vi "Measurement Logic.vi"(8 "error in":errorcluster, 9 "measurement configuration":T2={"Automation Test"=FALSE, "Power sequencing file path"="", "RFmx name"="5842_0", "RFmx port"="", "DUT Max Gain (dB)"=2.0, "DUT Max Noise Figure (dB)"=2.0, "Reference Level Mode"=enum."Manual", "Reference Level (dBm)"=2.0, "Preamp Enabled"=1, "RFmx attenuation mode"=enum."Constant Attenuation", "RFmx external attenuation (dB)"=1.2, "RFmx s-parameters orientation"=enum."Port2 Towards DUT", "RFmx s2p file path"="", "Switch Name"="", "Switch Connection"="", "ENS SMU Name"="", "ENS SMU Channel"="", "Action"=0, "Measurement Bandwidth (Hz)"=4000000.0, "Measurement Interval (s)"=0.1, "NF Cal Setup ID"="SNS_PS_6dB_ENR15_26.5GHz_VI", "DUT Type"=0, "Frequency List Mode"=enum."Step", "Step - Start Frequency "=1000000000.0, "Step - Stop Frequency"=2000000000.0, "Step - Step Size"=100000000.0, "Points - Start Frequency"=1000000000.0, "Points - Stop Frequency"=2000000000.0, "Points - Number of Points"=11, "FreqList - Frequency List"=[4000000000.0, 5000000000.0, 6000000000.0, 7000000000.0, 8000000000.0, 9000000000.0, 10000000000.0, 11000000000.0, 12000000000.0, 13000000000.0, 14000000000.0, 15000000000.0, 16000000000.0, 17000000000.0, 18000000000.0, 19000000000.0, 20000000000.0], "Averaging Enabled"=FALSE, "Averaging Count"=10, "Noise Source Type"=1, "Noise Source RFSG Port"="port1", "Noise Source Cold Temperature (K)"=302.8, "Noise Source Off Temperature (K)"=297.0, "ENR Freq (Hz)"=[6500000000.0], "ENR (dB)"=[15.0], "DUT Input_Compensation Enabled"=FALSE, "DUT Input_Temperation (K)"=297.0, "DUT Input_Loss Freq (Hz)"=array[589 elements], "DUT Input_Loss (dB)"=array[589 elements], "DUT Output_Compensation Enabled"=FALSE, "DUT Output_Temperation (K)"=297.0, "DUT Output_Loss Freq (Hz)"=array[589 elements], "DUT Output_Loss (dB)"=array[589 elements], "Calibration_Compensation Enabled"=FALSE, "Calibration_Temperation (K)"=297.0, "Calibration_Loss Freq (Hz)"=array[589 elements], "Calibration_Loss (dB)"=array[589 elements], "Noise Source_Compensation Enabled"=FALSE, "Noise Source_Temperation (K)"=297.0, "Noise Source_Loss Freq (Hz)"=[], "Noise Source_Loss (dB)"=[], "DUT Input Loss S2P File Path"="", "DUT Input Loss S-Parameter Orientation"=0, "DUT Output Loss S2P File Path"="", "DUT Output Loss S-Parameter Orientation"=0, "Calibration Loss S2P File Path"="", "Calibration Loss S-Parameter Orientation"=0, "Noise Source Loss S2P File Path"="", "Noise Source Loss S-Parameter Orientation"=0} {"Noise Source Loss S-Parameter Orientation" items=["Port1 Towards DUT", "Port2 Towards DUT"]; "Calibration Loss S-Parameter Orientation" items=["Port1 Towards DUT", "Port2 Towards DUT"]; "DUT Output Loss S-Parameter Orientation" items=["Port1 Towards DUT", "Port2 Towards DUT"]; "DUT Input Loss S-Parameter Orientation" items=["Port1 Towards DUT", "Port2 Towards DUT"]; "FreqList - Frequency List" format="%.3p Hz"; "Points - Stop Frequency" format="%.3p Hz"; "Points - Start Frequency" format="%.3p Hz"; "Step - Step Size" format="%.3p Hz"; "Step - Stop Frequency" format="%.3p Hz"; "Step - Start Frequency" format="%.3p Hz"; "Noise Source_Loss (dB)" format="%.2g"; "Noise Source_Loss Freq (Hz)" format="%.3p"; "Noise Source_Temperation (K)" format="%.2g"; "Calibration_Loss (dB)" format="%.2g"; "Calibration_Loss Freq (Hz)" format="%.3p"; "Calibration_Temperation (K)" format="%.2g"; "DUT Output_Loss (dB)" format="%.2g"; "DUT Output_Loss Freq (Hz)" format="%.3p"; "DUT Output_Temperation (K)" format="%.2g"; "DUT Input_Loss (dB)" format="%.2g"; "DUT Input_Loss Freq (Hz)" format="%.3p"; "DUT Input_Temperation (K)" format="%.2g"; "ENR (dB)" format="%.2g"; "ENR Freq (Hz)" format="%.3p"; "Noise Source Off Temperature (K)" format="%.2f"; "Noise Source Cold Temperature (K)" format="%.2f"; "Noise Source Type" items=["External Noise Source", "RF Signal Generator"]; "DUT Type" items=["Amplifier", "Downconverter", "Upconverter"]; "Measurement Interval (s)" format="%.2p"; "Measurement Bandwidth (Hz)" format="%.3p"; "Action" items=["Measure", "Calibrate"]; "RFmx external attenuation (dB)" format="%.2f"; "Preamp Enabled" items=["Disabled"=0, "Enabled"=1, "Automatic"=3]}, 10 "measure call context in":refnum<class "Measure Call Context.lvclass">) -> (0 "error out":errorcluster, 1 "measurement results":T1 {"Analyzer NF (mean)" format="%.2g"; "DUT NF (mean)" format="%.2g"; "Analyzer NF vs Freq" format="%.2g"; "DUT NF vs Freq" format="%.2g"}, 2 "measure call context out":refnum<class "Measure Call Context.lvclass">)   [LabVIEW 2023, in "FPT NoiseFigure.lvclass"]
doc: "Contains the core logic for executing the measurement."
uses:
  FPT NoiseFigure.lvclass
  <vilib>/Plug-In SDKs/Measurements/Measure Call Context/Measure Call Context.lvclass
  Measurement Configuration.ctl
  Measurement Results.ctl
  <vilib>/Analysis/baseanly.llb/Mean (DBL).vi
  <extravilib>/ChannelInstances/Event Messenger-bool/Instantiate.vi
  <vilib>/Analysis/NI_AALBase.lvlib
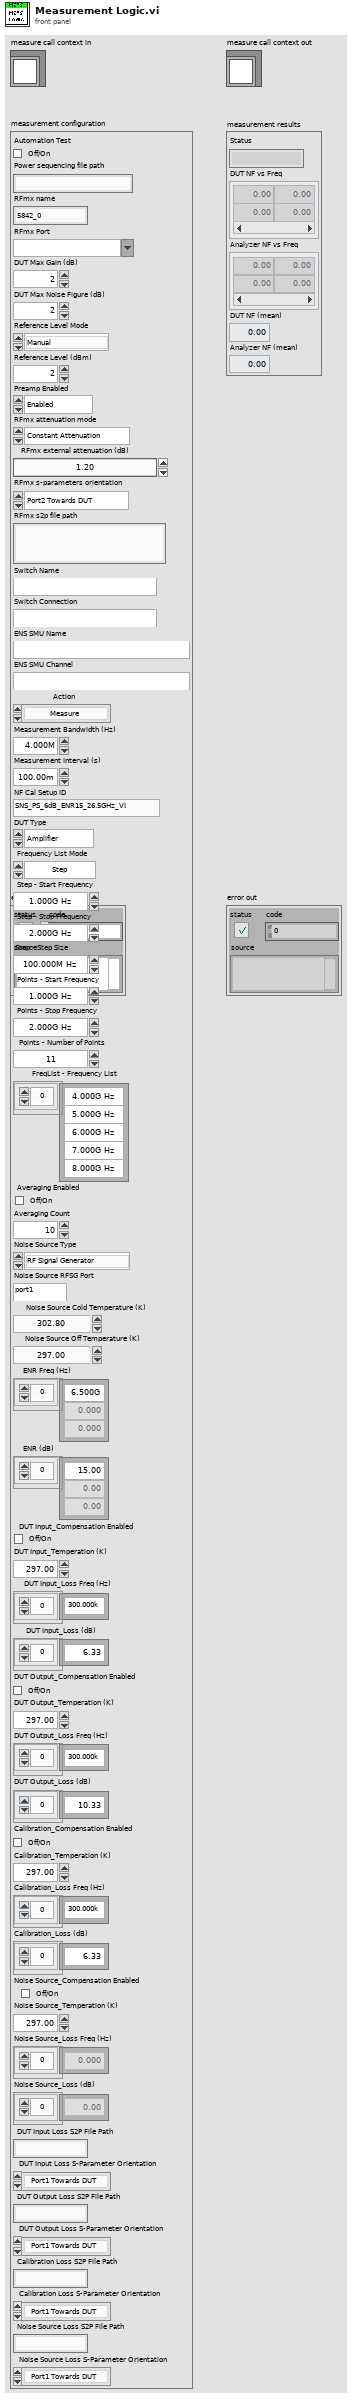
[diagram p1: front panel]
types:
  T1 = typedef "FPT NoiseFigure.lvclass/Measurement Results.ctl" = cluster{"Status":string, "DUT NF vs Freq":dbl[][], "Analyzer NF vs Freq":dbl[][], "DUT NF (mean)":dbl, "Analyzer NF (mean)":dbl}
  T2 = typedef "FPT NoiseFigure.lvclass/Measurement Configuration.ctl" = cluster{"Automation Test":bool, "Power sequencing file path":string, "RFmx name":string, "RFmx port":string, "DUT Max Gain (dB)":dbl, "DUT Max Noise Figure (dB)":dbl, "Reference Level Mode":enum32{"Manual", "Recommend"}, "Reference Level (dBm)":dbl, "Preamp Enabled":i32, "RFmx attenuation mode":enum32{"<None>", "Constant Attenuation", "s2p File"}, "RFmx external attenuation (dB)":dbl, "RFmx s-parameters orientation":enum32{"Port1 Towards DUT", "Port2 Towards DUT"}, "RFmx s2p file path":string, "Switch Name":string, "Switch Connection":string, "ENS SMU Name":string, "ENS SMU Channel":string, "Action":u32, "Measurement Bandwidth (Hz)":dbl, "Measurement Interval (s)":dbl, "NF Cal Setup ID":string, "DUT Type":i32, "Frequency List Mode":enum32{"Step", "Points", "Frequency List"}, "Step - Start Frequency ":dbl, "Step - Stop Frequency":dbl, "Step - Step Size":dbl, "Points - Start Frequency":dbl, "Points - Stop Frequency":dbl, "Points - Number of Points":i32, "FreqList - Frequency List":dbl[], "Averaging Enabled":bool, "Averaging Count":i32, "Noise Source Type":i32, "Noise Source RFSG Port":string, "Noise Source Cold Temperature (K)":dbl, "Noise Source Off Temperature (K)":dbl, "ENR Freq (Hz)":dbl[], "ENR (dB)":dbl[], "DUT Input_Compensation Enabled":bool, "DUT Input_Temperation (K)":dbl, "DUT Input_Loss Freq (Hz)":dbl[], "DUT Input_Loss (dB)":dbl[], "DUT Output_Compensation Enabled":bool, "DUT Output_Temperation (K)":dbl, "DUT Output_Loss Freq (Hz)":dbl[], "DUT Output_Loss (dB)":dbl[], "Calibration_Compensation Enabled":bool, "Calibration_Temperation (K)":dbl, "Calibration_Loss Freq (Hz)":dbl[], "Calibration_Loss (dB)":dbl[], "Noise Source_Compensation Enabled":bool, "Noise Source_Temperation (K)":dbl, "Noise Source_Loss Freq (Hz)":dbl[], "Noise Source_Loss (dB)":dbl[], "DUT Input Loss S2P File Path":string, "DUT Input Loss S-Parameter Orientation":i32, "DUT Output Loss S2P File Path":string, "DUT Output Loss S-Parameter Orientation":i32, "Calibration Loss S2P File Path":string, "Calibration Loss S-Parameter Orientation":i32, "Noise Source Loss S2P File Path":string, "Noise Source Loss S-Parameter Orientation":i32}
  T3 = enum32{"Power On Dut", "De-embedding + Measurement", "Power Off Dut"}[]
  T4 = cluster{"measurement configuration":T2, "measurement results":T1}
  T5 = typedef "RFmx Config - NF.ctl" = cluster{"RFmx Name":refnum<k15>, "RFmx Port":string, "Reference Level":cluster{"DUT Max Gain (dB)":dbl, "DUT Max Noise Figure (dB)":dbl, "Mode":enum32{"Manual", "Recommend"}, "Reference Level (dBm)":dbl}, "Preamp Enabled":i32, "Attenuation":cluster{"Mode":enum32{"<None>", "Constant Attenuation", "s2p File"}, "Constant Attenuation":cluster{"RFmx External Attenuation (dB)":dbl}, "s2p File":cluster{"RFmx S-Parameters Orientation":i32, "RFmx Attenuation s2p File":path}}, "ENS Source":cluster{"SMU Name":refnum<k15>, "SMU Channel":string}}
  T6 = typedef "Test Config - NF.ctl" = cluster{"Y-Factor Mode":i32, "Measurement Bandwidth (Hz)":dbl, "Measurement Interval (s)":dbl, "NF Cal Setup ID":string, "NF DUT Type":i32, "Frequency List (Hz)":dbl[], "Averaging":cluster{"Enabled":i32, "Count":i32}, "Noise Source":cluster{"Noise Source Type":i32, "Noise Source RFSG Port":string, "Cold Temperature (K)":dbl, "Off Temperature (K)":dbl, "ENR Freq (Hz)":dbl[], "ENR (dB)":dbl[]}}
  T7 = typedef "Switches - NF.ctl" = cluster{"Switch Name":refnum<k15>, "Connection":string}
  T8 = typedef "Path Loss Settings Cluster.ctl" = cluster{"DUT Input Loss":T9, "DUT Output Loss":T9, "Calibration Loss":T9, "Noise Source Loss":T9}
  T9 = typedef "Path Loss Settings.ctl" = cluster{"Compensation Enabled":i32, "Temperation (K)":dbl, "S2P Path":path, "Orientation":enum32{"Port1 Towards DUT", "Port2 Towards DUT"}}
  T10 = typedef "Event Messenger-bool.lvlib/))Channel.ctl" = refnum<queue>
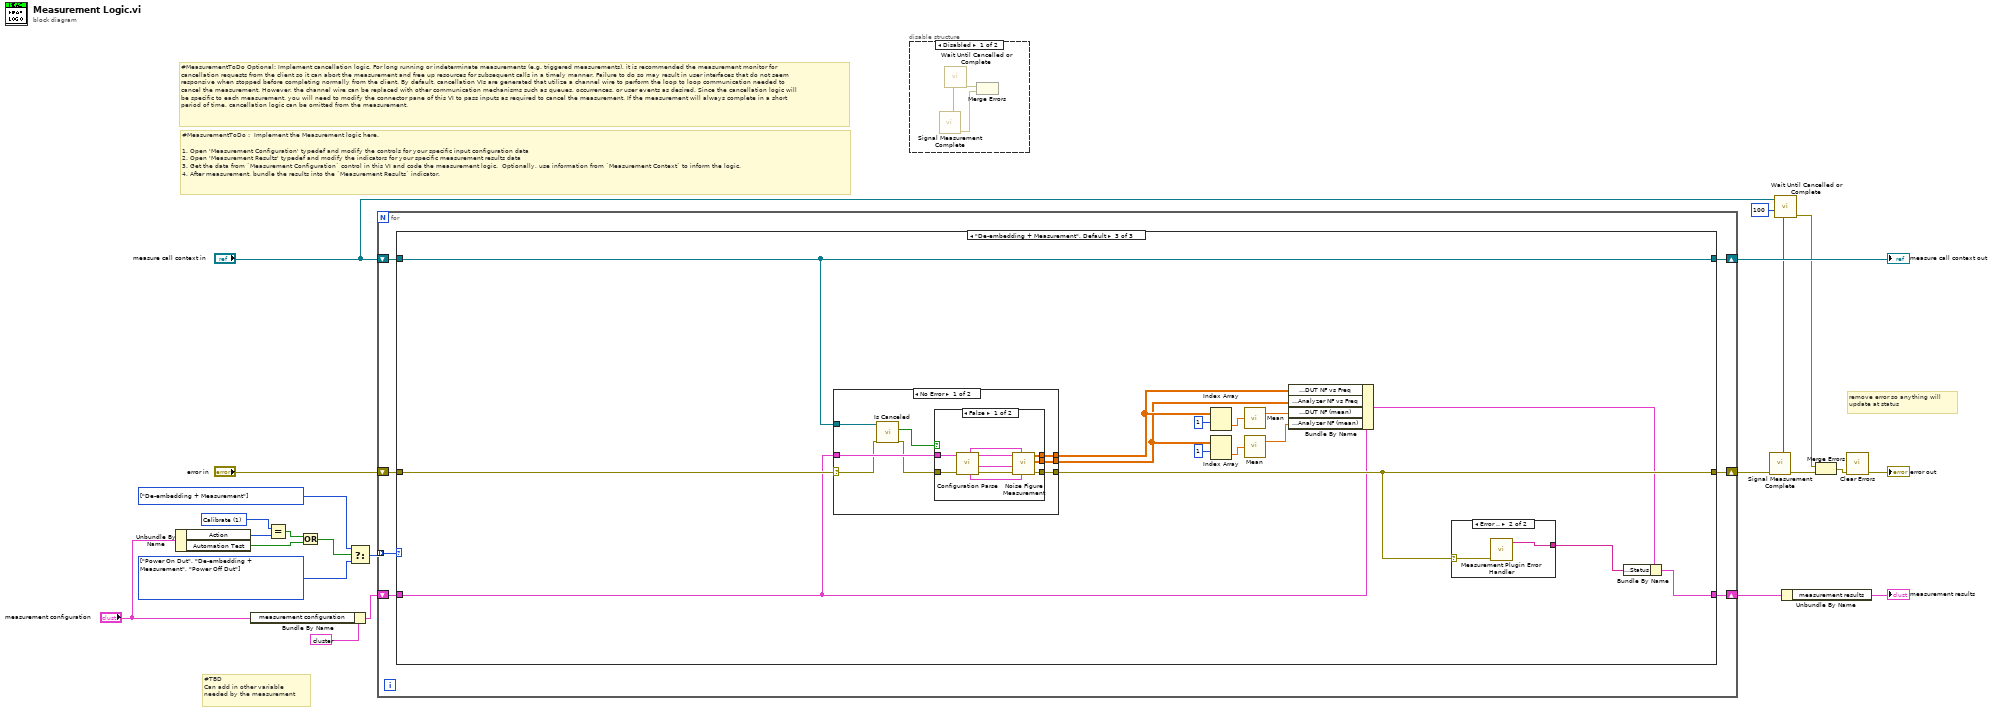
[diagram p0: block diagram]
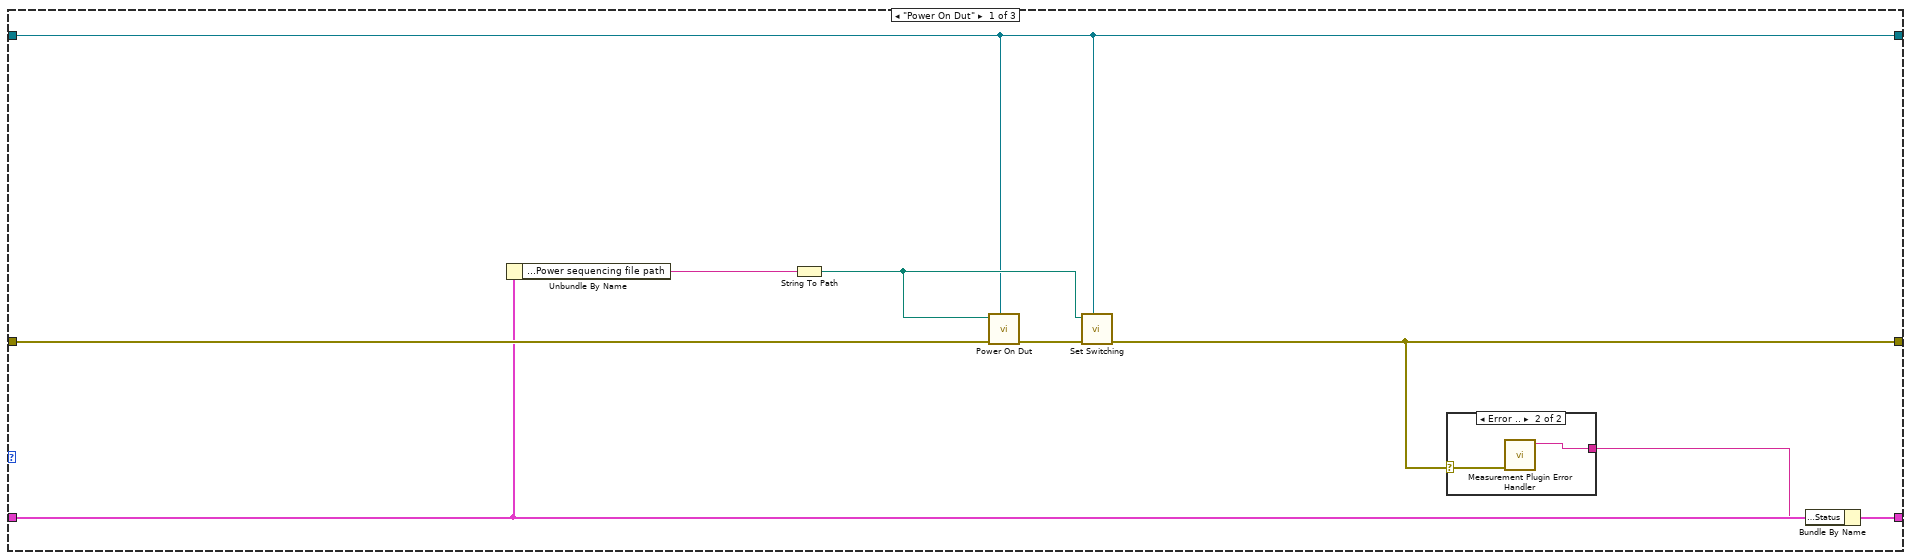
[diagram p2: hidden frame]
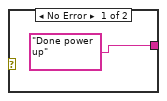
[diagram p3: hidden frame]
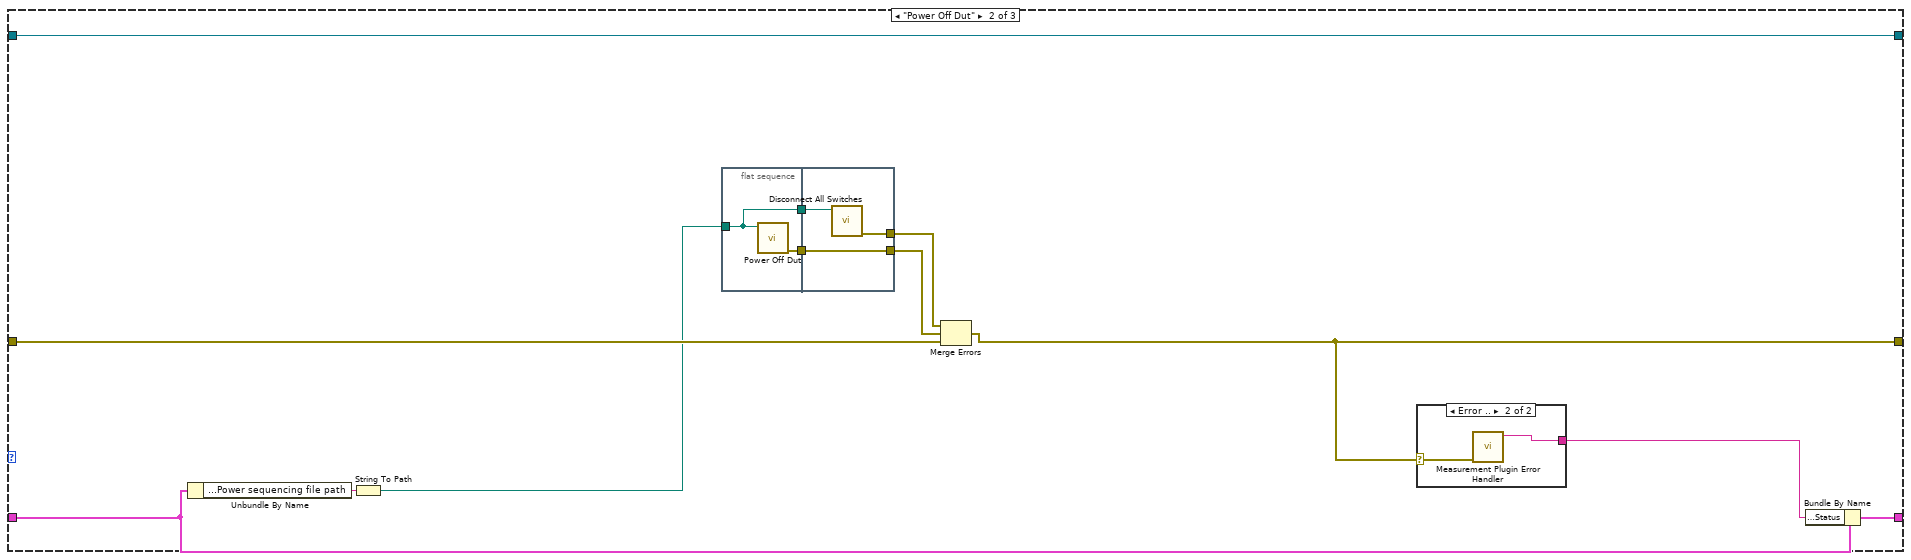
[diagram p4: hidden frame]
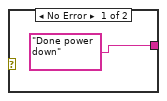
[diagram p5: hidden frame]
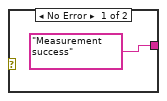
[diagram p6: hidden frame]
diagram:
  w8 = u32 1 items=["Measure", "Calibrate"] ("Y-Factor Mode")
  w15 = T3 [enum."De-embedding + Measurement"] items=["Power On Dut", "De-embedding + Measurement", "Power Off Dut"]
  w16 = T3 [enum."Power On Dut", enum."De-embedding + Measurement", enum."Power Off Dut"] items=["Power On Dut", "De-embedding + Measurement", "Power Off Dut"]
  # "remove error so anything will\nupdate at status"
  # "#TBD\nCan add in other variable\nneeded by the measurement"
  # "#MeasurementToDo Optional: Implement cancellation logic. For long running or indeterminate measurements (e.g. triggered measurements), it is recommended the measurement monitor for cancellation requests from the client so it can abort the measurement and free up resources for subsequent calls in a timely manner. Failure to do so may result in user interfaces that do not seem responsive when stopped before completing normally from the client. By default, cancellation VIs are generated that utilize a channel wire to perform the loop to loop communication needed to cancel the measurement. However, the channel wire can be replaced with other communication mechanisms such as queues, occurrences, or user events as desired. Since the cancellation logic will be specific to each measurement, you will need to modify the connector pane of this VI to pass inputs as required to cancel the measurement. If the measurement will always complete in a short period of time, cancellation logic can be omitted from the measurement."
  # "#MeasurementToDo :  Implement the Measurement logic here.\n\n1. Open 'Measurement Configuration' typedef and modify the controls for your specific input configuration data\n2. Open 'Measurement Results' typedef and modify the indicators for your specific measurement results data\n3. Get the data from `Measurement Configuration` control in this VI and code the measurement logic.  Optionally, use information from `Measurement Context` to inform the logic.\n4. After measurement, bundle the results into the `Measurement Results` indicator."
  n1 = Unbundle By Name("measurement configuration") -> ("Action"=w13:u32, "Automation Test"=w11:bool)
  n2 = Bundle By Name(cluster=T4 {"measurement configuration"={"Automation Test"=FALSE, "Power sequencing file path"="", "RFmx name"="5842_0", "RFmx port"="", "DUT Max Gain (dB)"=2.0, "DUT Max Noise Figure (dB)"=2.0, "Reference Level Mode"=enum."Manual", "Reference Level (dBm)"=2.0, "Preamp Enabled"=1, "RFmx attenuation mode"=enum."Constant Attenuation", "RFmx external attenuation (dB)"=1.2, "RFmx s-parameters orientation"=enum."Port2 Towards DUT", "RFmx s2p file path"="", "Switch Name"="", "Switch Connection"="", "ENS SMU Name"="", "ENS SMU Channel"="", "Action"=0, "Measurement Bandwidth (Hz)"=4000000.0, "Measurement Interval (s)"=0.1, "NF Cal Setup ID"="SNS_PS_6dB_ENR15_26.5GHz_VI", "DUT Type"=0, "Frequency List Mode"=enum."Step", "Step - Start Frequency "=1000000000.0, "Step - Stop Frequency"=2000000000.0, "Step - Step Size"=100000000.0, "Points - Start Frequency"=1000000000.0, "Points - Stop Frequency"=2000000000.0, "Points - Number of Points"=11, "FreqList - Frequency List"=[4000000000.0, 5000000000.0, 6000000000.0, 7000000000.0, 8000000000.0, 9000000000.0, 10000000000.0, 11000000000.0, 12000000000.0, 13000000000.0, 14000000000.0, 15000000000.0, 16000000000.0, 17000000000.0, 18000000000.0, 19000000000.0, 20000000000.0], "Averaging Enabled"=FALSE, "Averaging Count"=10, "Noise Source Type"=1, "Noise Source RFSG Port"="port1", "Noise Source Cold Temperature (K)"=302.8, "Noise Source Off Temperature (K)"=297.0, "ENR Freq (Hz)"=[6500000000.0], "ENR (dB)"=[15.0], "DUT Input_Compensation Enabled"=FALSE, "DUT Input_Temperation (K)"=297.0, "DUT Input_Loss Freq (Hz)"=array[589 elements], "DUT Input_Loss (dB)"=array[589 elements], "DUT Output_Compensation Enabled"=FALSE, "DUT Output_Temperation (K)"=297.0, "DUT Output_Loss Freq (Hz)"=array[589 elements], "DUT Output_Loss (dB)"=array[589 elements], "Calibration_Compensation Enabled"=FALSE, "Calibration_Temperation (K)"=297.0, "Calibration_Loss Freq (Hz)"=array[589 elements], "Calibration_Loss (dB)"=array[589 elements], "Noise Source_Compensation Enabled"=FALSE, "Noise Source_Temperation (K)"=297.0, "Noise Source_Loss Freq (Hz)"=[], "Noise Source_Loss (dB)"=[], "DUT Input Loss S2P File Path"="", "DUT Input Loss S-Parameter Orientation"=0, "DUT Output Loss S2P File Path"="", "DUT Output Loss S-Parameter Orientation"=0, "Calibration Loss S2P File Path"="", "Calibration Loss S-Parameter Orientation"=0, "Noise Source Loss S2P File Path"="", "Noise Source Loss S-Parameter Orientation"=0}, "measurement results"={"Status"="", "DUT NF vs Freq"=[], "Analyzer NF vs Freq"=[], "DUT NF (mean)"=0.0, "Analyzer NF (mean)"=0.0}}, "measurement configuration"="measurement configuration") -> (w21:T4)
  n3 = Equal?(x=w8, y=w13) -> (x = y?=w14:bool)
  n4 = Or(x=w14, y=w11) -> (x .or. y?=w12:bool)
  n5 = Select(t=w15, s=w12, f=w16) -> (s? t:f=w10:T3)
  n6 = for {
    tunnel: w10 -> [w29] mode=indexing
    shift-right: [w24] -> w5
    shift-left: "error in" -> [w30]
    shift-right: [w25] -> w19
    shift-left: w21 -> [w28]
    shift-right: [w26] -> w20
    shift-left: "measure call context in" -> [w27]
    n7 = case shown="\"De-embedding + Measurement\", Default" w29 {
      tunnel: w30 -> [w39 w49 w65]
      tunnel: w28 -> [w38 w50 w64]
      tunnel: w27 -> [w31 w53 w63]
      tunnel: [w33 w48 w75] -> w24
      tunnel: [w31 w53 w63] -> w26
      tunnel: [w36 w51 w76] -> w25
      frame "Power On Dut" {
        n8 = Unbundle By Name(w38) -> ("measurement configuration.Power sequencing file path"=w35:string)
        n9 = String To Path(string=w35) -> (path=w32:path)
        n10 = call "Power On Dut.vi"("measure call context in"=w31, "error in"=w39, "Power sequencing file path"=w32) -> ("error out"=w34:errorcluster)  [unwired: 7 in, 1 out]
        n11 = call "Set Switching.vi"("measure call context in"=w31, "error in"=w34, "File Path"=w32) -> ("error out"=w33:errorcluster)  [unwired: 7 in, 1 out]
        n12 = case shown="Error .." w33 {
          selector: w33 -> [_ w42]
          tunnel: ["Done power up" w41] -> w37
          frame No Error {
          }
          frame Error {
            n13 = call "Measurement Plugin Error Handler.vi"("error in"=w42) -> ("Status Message (Error)"=w41:string)  [unwired: 9 in, 1 out]
          }
        }
        n14 = Bundle By Name(cluster=w38, "measurement results.Status"=w37) -> (w36:T4)
      }
      frame "Power Off Dut" {
        n15 = Unbundle By Name(w50) -> ("measurement configuration.Power sequencing file path"=w54:string)
        n16 = String To Path(string=w54) -> (path=w45:path)
        n17 = flat-sequence {
          tunnel: w45 -> [w58]
          tunnel: [w59] -> w47
          tunnel: [w58] -> w46
          tunnel: [w62] -> w44
          tunnel: w47 -> [w62]
          tunnel: [w61] -> w43
          tunnel: w46 -> [w60]
          frame #0 {
            n18 = call "Power Off Dut.vi"("Power Sequencing File Path"=w58) -> ("error out"=w59:errorcluster)  [unwired: 10 in]
          }
          frame #1 {
            n19 = call "Disconnect All Switches.vi"("File Path"=w60) -> ("error out"=w61:errorcluster)  [unwired: 10 in]
          }
        }
        n20 = Merge Errors(w43, w44, w49) -> (w48:errorcluster)
        n21 = case shown="Error .." w48 {
          selector: w48 -> [_ w57]
          tunnel: ["Done power down" w56] -> w52
          frame No Error {
          }
          frame Error {
            n22 = call "Measurement Plugin Error Handler.vi"("error in"=w57) -> ("Status Message (Error)"=w56:string)  [unwired: 9 in, 1 out]
          }
        }
        n23 = Bundle By Name(cluster=w50, "measurement results.Status"=w52) -> (w51:T4)
      }
      frame "De-embedding + Measurement", Default {
        n24 = case shown="No Error" w65 {
          selector: w65 -> [w83 w100]
          tunnel: [w88 w100] -> w75
          tunnel: [w87 _] -> w67
          tunnel: [w86 _] -> w66
          tunnel: w64 -> [w85 _]
          tunnel: w63 -> [w82 _]
          frame No Error {
            n25 = call <vilib>:"Is Canceled.vi"("error in"=w83, "measure call context in"=w82) -> ("error out"=w84:errorcluster, "is canceled?"=w81:bool)  [unwired: 7 in, 1 out]
            n26 = case shown="False" w81 {
              tunnel: [w98 w99] -> w88
              tunnel: [w93 _] -> w87
              tunnel: [w92 _] -> w86
              tunnel: w85 -> [w90 _]
              tunnel: w84 -> [w89 w99]
              frame False {
                n27 = call "Configuration Parse.vi"("error in"=w89, "UI Controls"=w90) -> ("error out"=w94:errorcluster, "RFmx Settings"=w96:T5, "Test Configuration"=w97:T6, "Switch"=w91:T7, "Path Losses"=w95:T8)  [unwired: 5 in]
                n28 = call "Noise Figure Measurement.vi"("Switch"=w91, "Path Losses"=w95, "error in"=w94, "RFmx Settings"=w96, "Test Configuration"=w97) -> ("error out"=w98:errorcluster, "Analyzer Noise Figure (dB)"=w92:dbl[][], "DUT Noise Figure (dB)"=w93:dbl[][])  [unwired: 3 in, 1 out]
              }
              frame True {
              }
            }
          }
          frame Error {
          }
        }
        n29 = Index Array(array=w67, index (row)=1) -> (element=w72:dbl[])  [unwired: 1 in]
        n30 = Index Array(array=w66, index (row)=1) -> (element=w71:dbl[])  [unwired: 1 in]
        n31 = call-poly <vilib>:"Mean.vi"("X"=w72) -> ("mean"=w69:dbl)  [unwired: 1 out]
        n32 = call-poly <vilib>:"Mean.vi"("X"=w71) -> ("mean"=w68:dbl)  [unwired: 1 out]
        n33 = Bundle By Name(cluster=w64, "measurement results.DUT NF vs Freq"=w67, "measurement results.Analyzer NF vs Freq"=w66, "measurement results.DUT NF (mean)"=w69, "measurement results.Analyzer NF (mean)"=w68) -> (w74:T4)
        n34 = case shown="Error .." w75 {
          selector: w75 -> [_ w80]
          tunnel: ["Measurement success" w79] -> w77
          frame No Error {
          }
          frame Error {
            n35 = call "Measurement Plugin Error Handler.vi"("error in"=w80) -> ("Status Message (Error)"=w79:string)  [unwired: 9 in, 1 out]
          }
        }
        n36 = Bundle By Name(cluster=w74, "measurement results.Status"=w77) -> (w76:T4)
      }
    }
  }
  "measure call context out" <- w20
  n37 = disable-structure shown="Disabled" {
    frame Disabled {
      n38 = call "Signal Measurement Complete.vi"() -> ("error out"=w102:errorcluster, "done channel"=w103:T10)  [unwired: 10 in]
      n39 = call "Wait Until Cancelled or Complete.vi"("done channel"=w103) -> ("error out"=w101:errorcluster)  [unwired: 9 in, 1 out]
      n40 = Merge Errors(w101, w102) -> ()  [unwired: 1 out]
    }
    frame Enabled {
    }
  }
  n41 = call "Signal Measurement Complete.vi"("error in (no error)"=w5) -> ("error out"=w4:errorcluster, "done channel"=w3:T10)  [unwired: 9 in]
  n42 = call "Wait Until Cancelled or Complete.vi"("done channel"=w3, "ms polling interval"=100, "measure call context in"="measure call context in") -> ("error out"=w6:errorcluster)  [unwired: 7 in, 1 out]
  n43 = Unbundle By Name(w19) -> ("measurement results"=→"measurement results":T1)
  n44 = Merge Errors(w6, w4) -> (w7:errorcluster)
  n45 = call <vilib>:"Clear Errors.vi"("error in (no error)"=w7) -> ("error out"=→"error out":errorcluster)  [unwired: 5 in, 1 out]
